vi "STM Write Message.vi"   [LabVIEW 2015]
doc: "This VI writes a package of data to a remote computer. It prepends a meta data ID number to each packet. \n\nThe data must be passed in as a String. The calling VI is responsible for flattening the desired data to a string before passing it to this VI. \n\nCopyright 2015, 2016, 2017 National Instruments Corporation\n\nLicensed under the Apache License, Version 2.0 (the \"License\"); you may not use this file except in compliance with the License.\n\n You may obtain a copy of the License at\n\n http://www.apache.org/licenses/LICENSE-2.0\n\nUnless required by applicable law or agreed to in writing, software distributed under the License is distributed on an \"AS IS\" BASIS, WITHOUT WARRANTIES OR CONDITIONS OF ANY KIND, either express or implied.\n\nSee the License for the specific language governing permissions and limitations under the License."
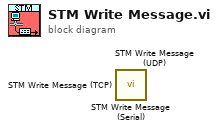
[diagram p0: block diagram]
diagram:
  n1 = call <vilib>:"STM Write Message (Serial).vi"() -> ()  [unwired: 10 in, 2 out]
  n2 = call <vilib>:"STM Write Message (UDP).vi"() -> ()  [unwired: 10 in, 2 out]
  n3 = call <vilib>:"STM Write Message (TCP).vi"() -> ()  [unwired: 10 in, 2 out]
